vi "Get Global VI Data.vi"(8 "error in (no error)":errorcluster, 11 "VI Ref":refnum<vi>) -> (0 "error out":errorcluster, 2 "VI Properties":T1, 3 "VI Ref out":refnum<vi>)   [LabVIEW 2020, in "VI Properties Editor.lvlib"]
doc: "Gets all data for a global VI."
uses:
  VI Properties Editor.lvlib
  <vilib>/picture/picture.llb/imagedata.ctl
  CTLs/VI Properties.ctl
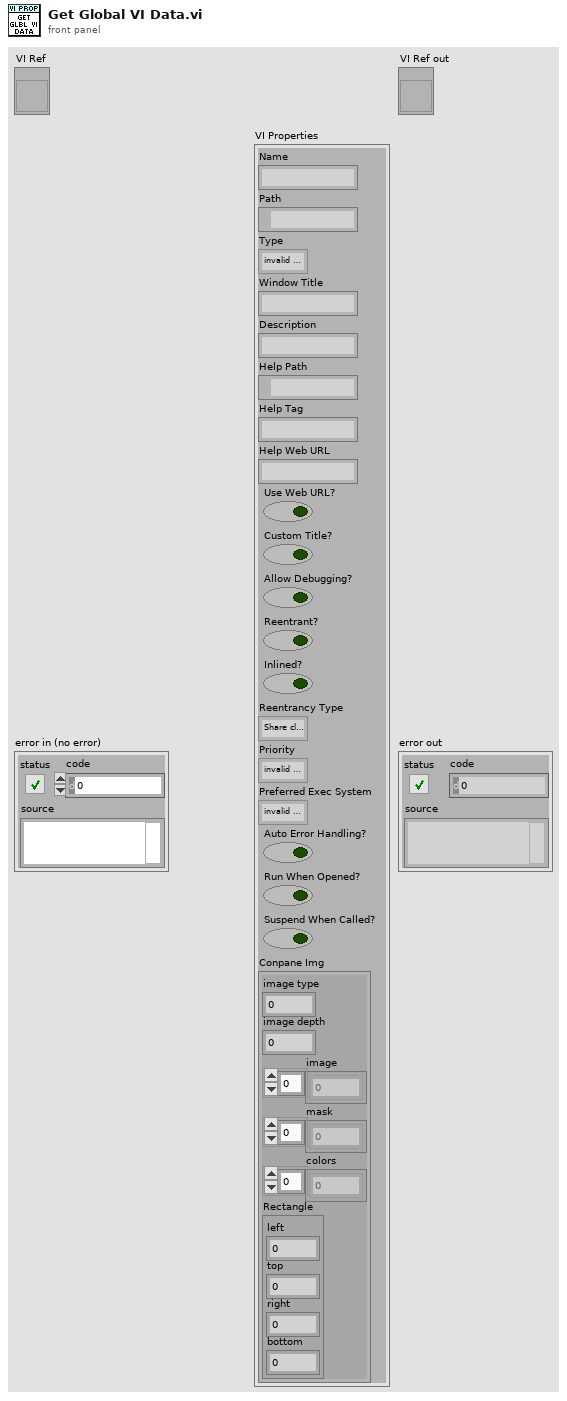
[diagram p1: front panel]
types:
  T1 = typedef "VI Properties Editor.lvlib/VI Properties.ctl" = cluster{"Name":string, "Path":path, "Type":enum32{"invalid VI type", "Standard VI", "Control VI", "Global VI", "Polymorphic VI", "Configuration VI", "SubSystem", "Facade VI", "Method VI", "Statechart Diagram VI"}, "Window Title":string, "Description":string, "Help Path":path, "Help Tag":string, "Help Web URL":string, "Use Web URL?":bool, "Custom Title?":bool, "Allow Debugging?":bool, "Reentrant?":bool, "Inlined?":bool, "Reentrancy Type":enum16{"Share clones between instances", "Preallocate clone for each instance"}, "Priority":enum32{"invalid priority", "background priority", "normal priority", "above normal priority", "high priority", "time critical priority", "subroutine"}, "Preferred Exec System":enum32{"invalid execution system", "user interface", "standard", "instrument i/o", "data acquisition", "other 1", "other 2", "same as caller"}, "Auto Error Handling?":bool, "Run When Opened?":bool, "Suspend When Called?":bool, "Conpane Img":T2}
  T2 = typedef "imagedata.ctl" = cluster{"image type":i32, "image depth":i32, "image":u8[], "mask":u8[], "colors":u32[], "Rectangle":cluster{"left":i16, "top":i16, "right":i16, "bottom":i16}}
  T3 = enum32{"invalid VI type", "Standard VI", "Control VI", "Global VI", "Polymorphic VI", "Configuration VI", "SubSystem", "Facade VI", "Method VI", "Statechart Diagram VI"}
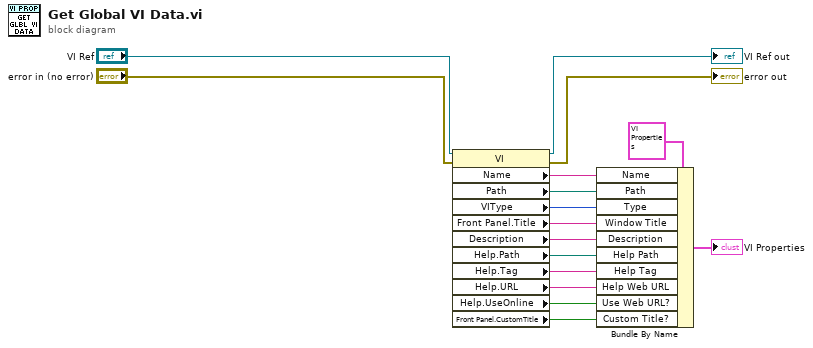
[diagram p0: block diagram]
diagram:
  n1 = property class="VI"(reference="VI Ref", error in="error in (no error)") -> (reference out=→"VI Ref out":refnum<vi>, error out=→"error out":errorcluster, "Name"=w15:string, "Path"=w14:path, "VIType"=w13:T3, "Front Panel.Title"=w4:string, "Description"=w12:string, "Help.Path"=w11:path, "Help.Tag"=w10:string, "Help.URL"=w2:string, "Help.UseOnline"=w1:bool, "Front Panel.CustomTitle"=w3:bool)
  n2 = Bundle By Name(cluster=T1 {"Name"="", "Path"=path "", "Type"=enum."invalid VI type", "Window Title"="", "Description"="", "Help Path"=path "", "Help Tag"="", "Help Web URL"="", "Use Web URL?"=FALSE, "Custom Title?"=FALSE, "Allow Debugging?"=FALSE, "Reentrant?"=FALSE, "Inlined?"=FALSE, "Reentrancy Type"=enum."Share clones between instances", "Priority"=enum."invalid priority", "Preferred Exec System"=enum."invalid execution system", "Auto Error Handling?"=FALSE, "Run When Opened?"=FALSE, "Suspend When Called?"=FALSE, "Conpane Img"={"image type"=0, "image depth"=0, "image"=[], "mask"=[], "colors"=[], "Rectangle"={"left"=0, "top"=0, "right"=0, "bottom"=0}}} ("VI Properties"), "Name"=w15, "Path"=w14, "Type"=w13, "Window Title"=w4, "Description"=w12, "Help Path"=w11, "Help Tag"=w10, "Help Web URL"=w2, "Use Web URL?"=w1, "Custom Title?"=w3) -> (→"VI Properties":T1)
